vi "Normalize 2D Array.vi"(1 "Array":dbl[][](array[numeric])=[[2.0, 1.0, 1.0, 0.0, 0.0], [1.0, 0.0, 0.0, 0.0, 0.0], [0.0, 0.0, 0.0, 0.0, 0.0], [3.0, 2.0, 1.0, 0.0, 0.0], [0.0, 0.0, 1.0, 3.0, 0.0]], 4 "Axis":u16(ring) items=["Rows", "Cols"]) -> (15 "Normalized":dbl[][](array[numeric])=[[0.3333333333333333, 0.3333333333333333, 0.3333333333333333, 0.0, 0.2], [0.16666666666666666, 0.0, 0.0, 0.0, 0.2], [0.0, 0.0, 0.0, 0.0, 0.2], [0.5, 0.6666666666666666, 0.3333333333333333, 0.0, 0.2], [0.0, 0.0, 0.3333333333333333, 1.0, 0.2]] format="%.2f", 18 "Sums":dbl[](array[numeric])=[6.0, 3.0, 3.0, 3.0, 0.0])   [LabVIEW 2014]
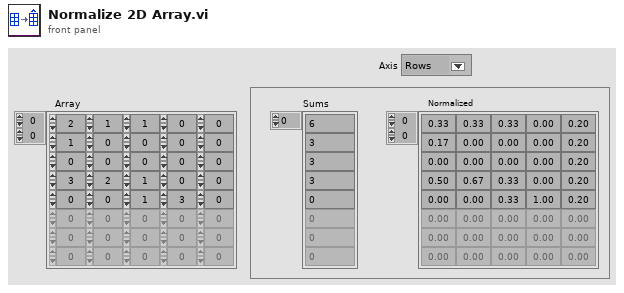
[diagram p1: front panel]
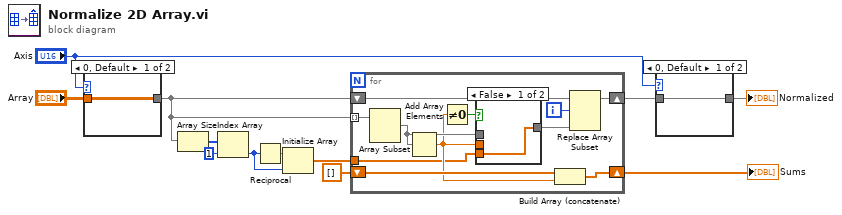
[diagram p0: block diagram]
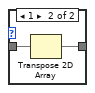
[diagram p2: hidden frame]
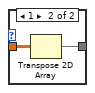
[diagram p3: hidden frame]
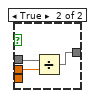
[diagram p4: hidden frame]
diagram:
  n1 = case shown="0, Default" "Axis" {
    tunnel: "Array" -> [w13 w15]
    tunnel: [w13 w14] -> w6
    frame 0, Default {
    }
    frame 1 {
      n2 = Transpose 2D Array(2D array=w15) -> (transposed array=w14:dbl[][])
    }
  }
  n3 = Array Size(array=w6) -> (size(s)=w5:i32[])
  n4 = Index Array(array=w5, index=1) -> (element=w2:i32)
  n5 = Reciprocal(x=w2) -> (1/x=w3:dbl)
  n6 = Initialize Array(w3, w2) -> (w1:dbl[])
  n7 = for {
    tunnel: w6 -> [w26] mode=indexing
    shift-right: [w25] -> w12
    shift-left: dbl[] [] -> [w24]
    shift-right: [w20] -> w9
    shift-left: w6 -> [w19]
    tunnel: w1 -> [w16]
    i -> [w22]
    n8 = Array Subset(array=w26) -> (w23:dbl[])  [unwired: 2 in]
    n9 = Add Array Elements(numeric array=w23) -> (sum=w17:dbl)
    n10 = Not Equal To 0?(x=w17) -> (x != 0?=w18:bool)
    n11 = case shown="False" w18 {
      tunnel: w23 -> [_ w30]
      tunnel: [w27 w29] -> w21
      tunnel: w17 -> [_ w28]
      tunnel: w16 -> [w27 _]
      frame False {
      }
      frame True {
        n12 = Divide(x=w30, y=w28) -> (x/y=w29:dbl[])
      }
    }
    n13 = Build Array (concatenate)(w24, w17) -> (w25:dbl[])
    n14 = Replace Array Subset(array=w19, new element=w21, index (row)=w22) -> (w20:dbl[][])  [unwired: 1 in]
  }
  "Sums" <- w12
  n15 = case shown="0, Default" "Axis" {
    tunnel: w9 -> [w31 w33]
    tunnel: [w31 w32] -> w8
    frame 0, Default {
    }
    frame 1 {
      n16 = Transpose 2D Array(2D array=w33) -> (transposed array=w32:dbl[][])
    }
  }
  "Normalized" <- w8
